vi "Initialize.vi"(4 "id":string, 6 "Path Transform":string, 8 "error in (no error)":errorcluster, 9 "Path Style":string, 10 "Path Data":string, 11 "Path in":refnum<class "Path.lvclass">) -> (0 "error out":errorcluster, 3 "Path out":refnum<class "Path.lvclass">)   [LabVIEW 2019, in "Path.lvclass"]
uses:
  Path.lvclass
  PathTokenizer/PathTokenizer.lvclass
  CSSProperties/CSSProperties.lvclass
  TransformTokenizer/TransformTokenizer.lvclass
  Path.lvclass/Path.ctl
  TransformTokenizer/TransformTokenizer.lvclass/TransformTokenizer.ctl
  Transform/Transform.lvclass
  Transform.Matrix/Transform.Matrix.lvclass
  C:/Users/Albro/Documents/GitHub/AFM-Lithography/lvsrc/Classes/Parse/Transform/Transform.lvclass
  Transform.Translate/Transform.Translate.lvclass
  Transform.Rotate/Transform.Rotate.lvclass
  Transform.Skew/Transform.Skew.lvclass
  PathTokenizer/PathTokenizer.lvclass/PathTokenizer.ctl
  PathCommands/PathCommands.lvclass
  PathCommands.Moveto/PathCommands.MoveTo.lvclass
  C:/Users/Albro/Documents/GitHub/AFM-Lithography/lvsrc/Classes/Parse/PathCommands/PathCommands.lvclass
  PathCommands.LineTo/PathCommands.LineTo.lvclass
  PathCommands.CurveTo/PathCommands.CurveTo.lvclass
  PathCommands.ClosePath/PathCommands.ClosePath.lvclass
  Write Path Commands.vi
  Write Transforms.vi
  Transform.Scale/Transform.Scale.lvclass
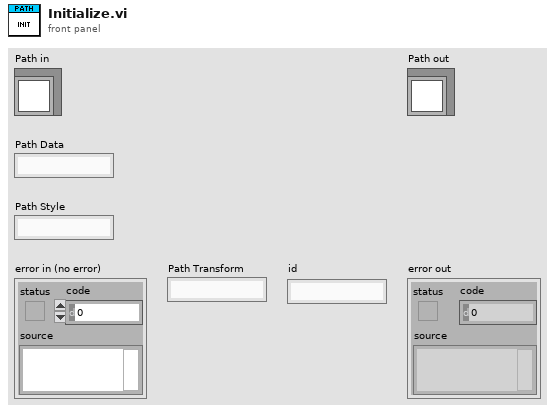
[diagram p1: front panel]
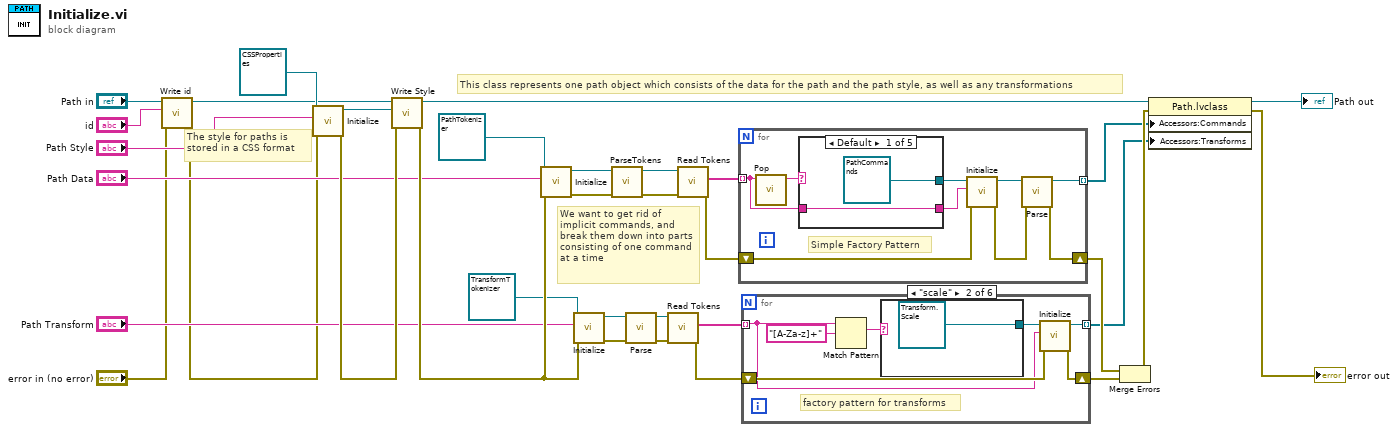
[diagram p0: block diagram]
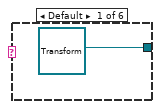
[diagram p2: hidden frame]
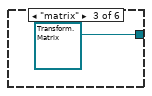
[diagram p3: hidden frame]
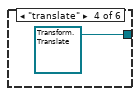
[diagram p4: hidden frame]
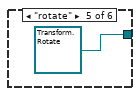
[diagram p5: hidden frame]
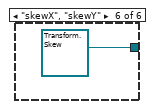
[diagram p6: hidden frame]
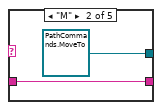
[diagram p7: hidden frame]
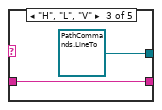
[diagram p8: hidden frame]
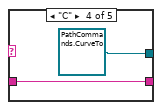
[diagram p9: hidden frame]
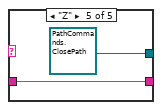
[diagram p10: hidden frame]
diagram:
  # "This class represents one path object which consists of the data for the path and the path style, as well as any transformations"
  # "We want to get rid of implicit commands, and break them down into parts consisting of one command at a time"
  # "The style for paths is stored in a CSS format"
  n1 = call-dynamic "Write id.vi"("error in (no error)"="error in (no error)", "id"="id", "SVG Object in"="Path in") -> ("error out"=w1:errorcluster, "SVG Object out"=w4:refnum<class "Path.lvclass">)  [unwired: 7 in]
  n2 = call "Initialize.vi"("error in (no error)"=w1, "Properties String"="Path Style", "CSSProperties in"=refnum<class "CSSProperties.lvclass"> refnum) -> ("error out"=w31:errorcluster, "CSSProperties out"=w15:refnum<class "CSSProperties.lvclass">)  [unwired: 7 in]
  n3 = call "Write Style.vi"("error in (no error)"=w31, "CSSProperties.lvclass"=w15, "Path in"=w4) -> ("error out"=w28:errorcluster, "Path out"=w8:refnum<class "Path.lvclass">)  [unwired: 7 in]
  n4 = call "Initialize.vi"("error in (no error)"=w28, "Path Command Text"="Path Data", "PathTokenizer in"=refnum<class "PathTokenizer.lvclass"> refnum ("PathTokenizer.lvclass")) -> ("error out"=w34:errorcluster, "PathTokenizer out"=w22:refnum<class "PathTokenizer.lvclass">)  [unwired: 7 in]
  n5 = call "Initialize.vi"("error in (no error)"=w28, "Transform Attribute String"="Path Transform", "TransformTokenizer in"=refnum<class "TransformTokenizer.lvclass"> refnum) -> ("error out"=w30:errorcluster, "TransformTokenizer out"=w14:refnum<class "TransformTokenizer.lvclass">)  [unwired: 7 in]
  n6 = call "ParseTokens.vi"("error in (no error)"=w34, "PathTokenizer in"=w22) -> ("error out"=w33:errorcluster, "PathTokenizer out"=w21:refnum<class "PathTokenizer.lvclass">)  [unwired: 8 in]
  n7 = call "Parse.vi"("error in (no error)"=w30, "TransformTokenizer in"=w14) -> ("error out"=w29:errorcluster, "TransformTokenizer out"=w11:refnum<class "TransformTokenizer.lvclass">)  [unwired: 8 in]
  n8 = call "Read Tokens.vi"("error in (no error)"=w29, "TransformTokenizer in"=w11) -> ("error out"=w27:errorcluster, "Transforms"=w10:string[])  [unwired: 7 in, 1 out]
  n9 = call "Read Tokens.vi"("error in (no error)"=w33, "PathTokenizer in"=w21) -> ("error out"=w32:errorcluster, "Tokens"=w19:string[])  [unwired: 7 in, 1 out]
  n10 = for {
    tunnel: w19 -> [w39] mode=indexing
    shift-right: [w41] -> w26
    shift-left: w32 -> [w43]
    tunnel: [w35] -> w7 mode=indexing
    # "Simple Factory Pattern"
    n11 = call "Pop.vi"("Command Text"=w39) -> ("Command Type"=w40:string)  [unwired: 9 in, 1 out]
    n12 = case shown="Default" w40 {
      tunnel: [refnum<class "PathCommands.lvclass"> refnum ("PathCommands.lvclass") refnum<class "PathCommands.MoveTo.lvclass"> refnum ("PathCommands.MoveTo.lvclass") refnum<class "PathCommands.LineTo.lvclass"> refnum ("PathCommands.LineTo.lvclass") refnum<class "PathCommands.CurveTo.lvclass"> refnum ("PathCommands.CurveTo.lvclass") refnum<class "PathCommands.ClosePath.lvclass"> refnum ("PathCommands.ClosePath.lvclass")] -> w38
      tunnel: [w44 w47 w49 w51 w53] -> w37
      tunnel: w39 -> [w44 w47 w49 w51 w53]
      frame Default {
      }
      frame "M" {
      }
      frame "H", "L", "V" {
      }
      frame "C" {
      }
      frame "Z" {
      }
    }
    n13 = call-dynamic "Initialize.vi"("error in (no error)"=w43, "CommandText"=w37, "PathCommands in"=w38) -> ("error out"=w42:errorcluster, "PathCommands out"=w36:refnum<class "PathCommands.lvclass">)  [unwired: 7 in]
    n14 = call-dynamic "Parse.vi"("error in (no error)"=w42, "PathCommands in"=w36) -> ("error out"=w41:errorcluster, "PathCommands out"=w35:refnum<class "PathCommands.lvclass">)  [unwired: 8 in]
  }
  n15 = for {
    tunnel: w10 -> [w54] mode=indexing
    shift-right: [w56] -> w25
    shift-left: w27 -> [w57]
    tunnel: [w55] -> w6 mode=indexing
    # "factory pattern for transforms"
    n16 = Match Pattern(string=w54, regular expression="[A-Za-z]+") -> (match substring=w59:string)  [unwired: 1 in, 3 out]
    n17 = case shown="\"scale\"" w59 {
      tunnel: [refnum<class "Transform.lvclass"> refnum ("Transform in") refnum<class "Transform.Scale.lvclass"> refnum ("Transform.Scale.lvclass") refnum<class "Transform.Matrix.lvclass"> refnum ("Transform.Matrix.lvclass") refnum<class "Transform.Translate.lvclass"> refnum ("Transform.Translate.lvclass") refnum<class "Transform.Rotate.lvclass"> refnum ("Transform.Rotate.lvclass") refnum<class "Transform.Skew.lvclass"> refnum ("Transform.Skew.lvclass")] -> w58
      frame Default {
      }
      frame "scale" {
      }
      frame "matrix" {
      }
      frame "translate" {
      }
      frame "rotate" {
      }
      frame "skewX", "skewY" {
      }
    }
    n18 = call-dynamic "Initialize.vi"("error in (no error)"=w57, "Transform"=w54, "Transform in"=w58) -> ("error out"=w56:errorcluster, "Transform out"=w55:refnum<class "Transform.lvclass">)  [unwired: 7 in]
  }
  n19 = Merge Errors(w26, w25) -> (w24:errorcluster)
  n20 = property class="Path.lvclass"(reference=w8, error in=w24, "Accessors:Commands"=w7, "Accessors:Transforms"=w6) -> (reference out=→"Path out":refnum<class "Path.lvclass">, error out=→"error out":errorcluster)
